vi "temperatura_termometro_grafico.vi"() -> ()   [LabVIEW 2018]
uses:
  <vilib>/Instr/_visa.llb/VISA Configure Serial Port (Instr).vi
panel:
  in  "Arquivo":path
  in  "?":bool
  out "?":bool
  in  "?":bool
  in  "VISA resource name":refnum<visa-resource-name>
  out "Thermometer":dbl(slide) scale=0.0..100.0
  out "Waveform Chart":i32(graph)
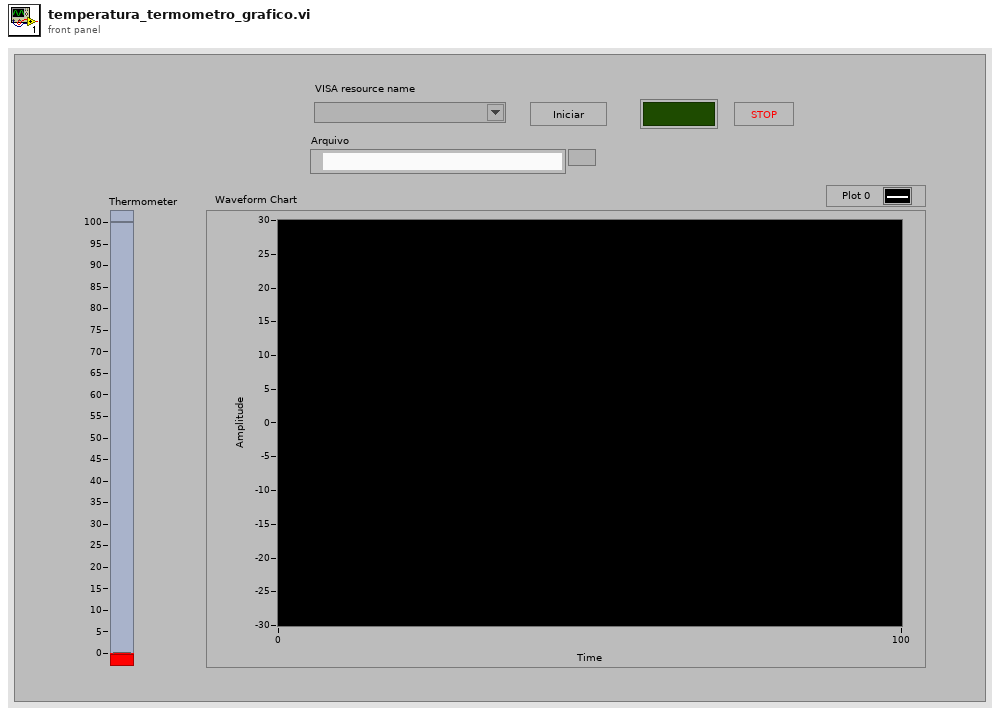
[diagram p1: front panel]
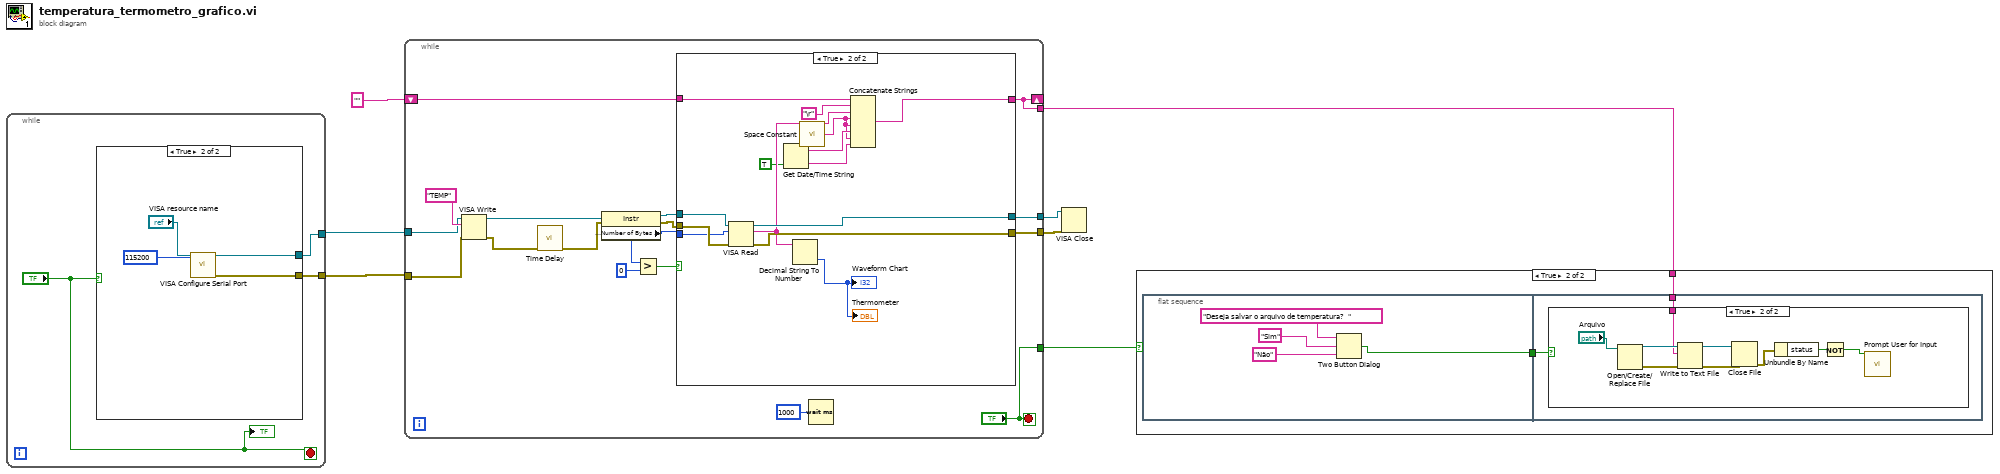
[diagram p0: block diagram]
diagram:
  n1 = while {
    tunnel: [w10] -> w6
    tunnel: [w9] -> w7
    stop <- "?" stop-if-true
    n2 = case shown="True" "?" {
      tunnel: [_ w12] -> w10
      tunnel: [_ w11] -> w9
      frame False {
      }
      frame True {
        n3 = call-poly "VISA Configure Serial Port"("VISA resource name"="VISA resource name", "baud rate (9600)"=u32 115200) -> ("VISA resource name out"=w12:refnum<visa-resource-name>, "error out"=w11:errorcluster)  [unwired: 12 in]
      }
    }
    "?" <- "?"
  }
  n4 = while {
    tunnel: w6 -> [w30]
    tunnel: w7 -> [w29]
    shift-right: [w15] -> _
    shift-left: "" -> [w20]
    tunnel: [w19] -> w4
    tunnel: [w18] -> w3
    tunnel: ["?"] -> w2
    tunnel: [w15] -> w1
    stop <- "?" stop-if-true
    n5 = VISA Write(VISA resource name=w30, write buffer="TEMP", error in (no error)=w29) -> (VISA resource name out=w27:refnum<visa-resource-name>, error out=w28:errorcluster)  [unwired: 1 out]
    n6 = call "Time Delay"("error in (no error)"=w28) -> ("error out"=w26:errorcluster)  [unwired: 10 in]
    n7 = property class="Instr"(reference=w27, error in=w26) -> (reference out=w23:refnum<visa-resource-name>, error out=w22:errorcluster, "Serial Settings:Number of Bytes at Serial Port"=w21:u32)
    n8 = Greater?(x=w21, y=u32 0) -> (0:w25:bool)
    n9 = case shown="True" w25 {
      tunnel: w23 -> [w34 w48]
      tunnel: w22 -> [w33 w47]
      tunnel: w21 -> [_ w46]
      tunnel: [w34 w45] -> w19
      tunnel: [w33 w44] -> w18
      tunnel: [w32 w35] -> w15
      tunnel: w20 -> [w32 w42]
      frame False {
      }
      frame True {
        n10 = VISA Read(VISA resource name=w48, byte count=w46, error in (no error)=w47) -> (VISA resource name out=w45:refnum<visa-resource-name>, read buffer=w40:string, error out=w44:errorcluster)  [unwired: 1 out]
        n11 = Get Date/Time String(want seconds? (F)=TRUE) -> (date string=w39:string, time string=w37:string)  [unwired: 2 in]
        n12 = Decimal String To Number(string=w40) -> (number=→"Waveform Chart" →"Thermometer":i32)  [unwired: 2 in, 1 out]
        n13 = call <vilib>:"Space Constant.vi"() -> ("String"=w38:string)
        n14 = Concatenate Strings(w42, "\r", w40, w38, w38, w39, w38, w37) -> (w35:string)
      }
    }
    n15 = Wait (ms)(milliseconds to wait=u32 1000) -> ()  [unwired: 1 out]
  }
  n16 = VISA Close(VISA resource name=w4, error in (no error)=w3) -> ()  [unwired: 1 out]
  n17 = case shown="True" w2 {
    tunnel: w1 -> [_ w50]
    frame False {
    }
    frame True {
      n18 = flat-sequence {
        tunnel: [w51] -> w49
        tunnel: w50 -> [w56]
        tunnel: w49 -> [w55]
        frame #0 {
          n19 = Two Button Dialog(message="Deseja salvar o arquivo de temperatura?  ", 1:"Não" ("F button name (\"Cancel\")"), 2:"Sim" ("T button name (\"OK\")")) -> (T button?=w51:bool)
        }
        frame #1 {
          n20 = case shown="True" w55 {
            tunnel: w56 -> [_ w62]
            frame False {
            }
            frame True {
              n21 = Open/Create/Replace File(file path (use dialog)="Arquivo") -> (refnum out=w64:refnum<file>, error out=w63:errorcluster)  [unwired: 5 in, 1 out]
              n22 = Write to Text File(file (use dialog)=w64, text=w62, error in=w63) -> (refnum out=w61:refnum<file>, error out=w60:errorcluster)  [unwired: 1 in, 1 out]
              n23 = Close File(refnum=w61, error in=w60) -> (error out=w59:errorcluster)  [unwired: 1 out]
              n24 = Unbundle By Name(w59) -> ("status"=w58:bool)
              n25 = Not(x=w58) -> (.not. x?=w57:bool)
              n26 = call "Prompt User for Input"("Enable"=w57) -> ()  [unwired: 17 in, 2 out]
            }
          }
        }
      }
    }
  }
